vi "Heapsort Test.vi"() -> ()   [LabVIEW 2018]
uses:
  543125ef-4f9d-45e7-86eb-6cd3a2813603.vi
  76c11280-2fa5-4099-b1d0-22009f2edf91.vi
  baa485c2-40bf-4992-8974-7a4648b610c0.vi
  543125ef-4f9d-45e7-86eb-6cd3a2813603.vi/56c2d4e2-0f90-4ccb-81e2-1783ffecbf3c.vi
  76c11280-2fa5-4099-b1d0-22009f2edf91.vi/cf578f05-2cb7-4387-8c8b-80cdb072d34e.vi
  baa485c2-40bf-4992-8974-7a4648b610c0.vi/bf8f5b7a-e52f-45c2-a695-8a4591f38db5.vi
  baa485c2-40bf-4992-8974-7a4648b610c0.vi/956c8940-c20a-4fa0-b644-bb8ca14a28e4.vi
  baa485c2-40bf-4992-8974-7a4648b610c0.vi/5a6b6c26-5945-41fa-9292-4092f6cf429a.vi
  baa485c2-40bf-4992-8974-7a4648b610c0.vi/bc6b2db0-348e-4cc1-97c1-9078f9776a65.vi
  baa485c2-40bf-4992-8974-7a4648b610c0.vi/bf8f5b7a-e52f-45c2-a695-8a4591f38db5.vi/c8fd2a1f-e26a-45fa-9413-b4f5b095b4bd.vi
  baa485c2-40bf-4992-8974-7a4648b610c0.vi/5a6b6c26-5945-41fa-9292-4092f6cf429a.vi/2bfd5eb4-be0b-4c91-969d-d1e0730fcb27.vi
  Shared/Graham Scan/Heapsort/Numeric Heapify.vi
panel:
  out "Sorted":cluster{i32[], "Range(st, stp, inc)":i32[]}(graph)
  out "Unsorted":T1(graph)
  in  "Number of Values":i32
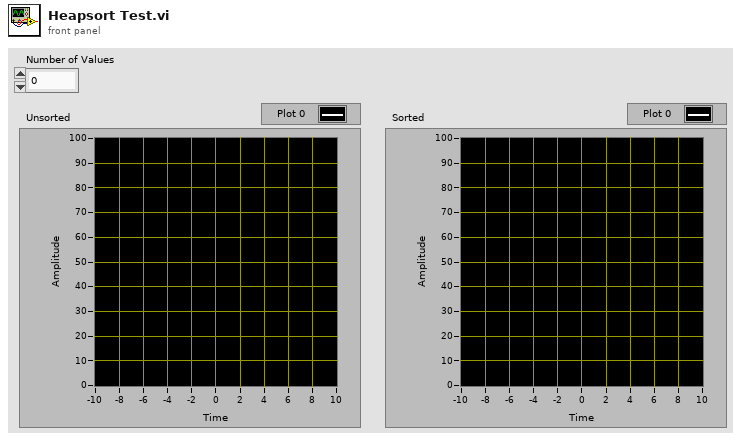
[diagram p1: front panel]
types:
  T1 = cluster{"Random Array":i32[], "Range(st, stp, inc)":i32[]}
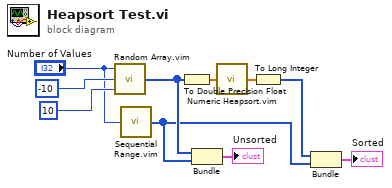
[diagram p0: block diagram]
diagram:
  n1 = call "Random Array.vim"("Max. (1, inc.)"=10, "Min. (0, inc.)"=-10, "Number of Elements (100)"="Number of Values") -> ("Random Array"=w7:i32[])
  n2 = call "Sequential Range.vim"("Stop (exc.)"="Number of Values") -> ("Range(st, stp, inc)"=w4:i32[])  [unwired: 2 in]
  n3 = To Double Precision Float(number=w7) -> (double precision float=w1:dbl[])
  n4 = Bundle("Random Array"=w7, "Range(st, stp, inc)"=w4) -> (→"Unsorted":T1)  [unwired: 1 in]
  n5 = call "Numeric Heapsort.vim"("Array"=w1) -> ("Sorted Array"=w5:dbl[])
  n6 = To Long Integer(number=w5) -> (32bit integer=w2:i32[])
  n7 = Bundle(w2, "Range(st, stp, inc)"=w4) -> (→"Sorted":cluster{i32[], "Range(st, stp, inc)":i32[]})  [unwired: 1 in]
